vi "Set_CleanCycleHeight.vi"(8 "error in":errorcluster, 10 "CleanCycleHeight":i32, 11 "camera handle in":u64) -> (0 "error out":errorcluster, 3 "camera handle out":u64)   [LabVIEW 2014, in "PICam.lvlib"]
doc: "Controls the number of rows in a clean cycle. The default value is equal with the Y pixel size of the CCD (for example, PIXIS400: 400)."
uses:
  PICam.lvlib
  Picam32.dll
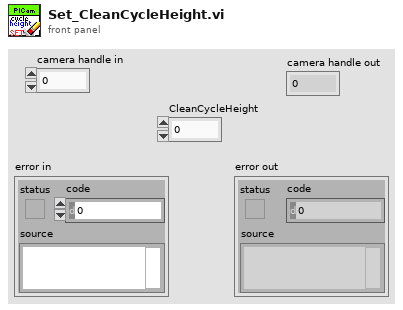
[diagram p1: front panel]
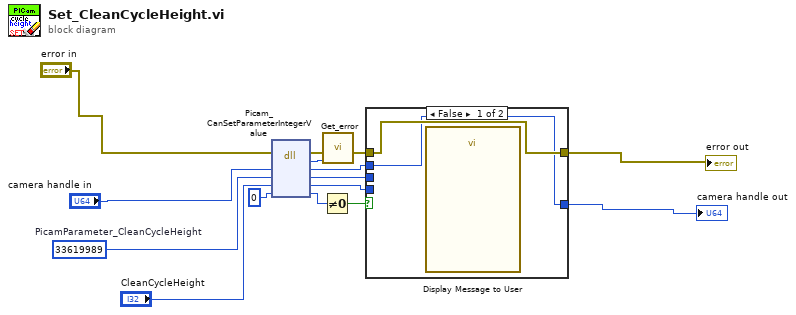
[diagram p0: block diagram]
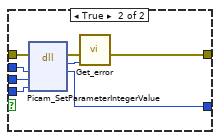
[diagram p2: hidden frame]
diagram:
  w6 = u32 33619989  # PicamParameter_CleanCycleHeight
  n1 = dll-call lib="Picam32.dll" fn="Picam_CanSetParameterIntegerValue"(error in="error in", "camera"="camera handle in", "PicamParameter"=w6, "CleanCycleHeight"="CleanCycleHeight", "bln"=0 ("CleanSerialRegister")) -> (error out=w14:errorcluster, "return type"=w15:i32, "camera"=w7:u64, "PicamParameter"=w5:u32, "CleanCycleHeight"=w10:i32, "bln"=w11:i32)  [unwired: 2 in, 1 out]
  n2 = Not Equal To 0?(x=w11) -> (x != 0?=w9:bool)
  n3 = call "Get_error.vi"("PICam_Error"=w15, "error in (no error)"=w14) -> ("error out"=w8:errorcluster)  [unwired: 9 in]
  n4 = case shown="False" w9 {
    tunnel: w10 -> [_ w23]
    tunnel: w8 -> [w17 w22]
    tunnel: w7 -> [w16 w21]
    tunnel: w5 -> [_ w20]
    tunnel: [w17 w19] -> w4
    tunnel: [w16 w18] -> w3
    frame False {
      n5 = call "Display Message to User"() -> ()  [unwired: 10 in, 2 out]
    }
    frame True {
      n6 = dll-call lib="Picam32.dll" fn="Picam_SetParameterIntegerValue"(error in=w22, "camera"=w21, "PicamParameter"=w20, "CleanCycleHeight"=w23) -> (error out=w25:errorcluster, "return type"=w24:i32, "camera"=w18:u64)  [unwired: 4 in, 1 out]
      n7 = call "Get_error.vi"("PICam_Error"=w24, "error in (no error)"=w25) -> ("error out"=w19:errorcluster)  [unwired: 9 in]
    }
  }
  "error out" <- w4
  "camera handle out" <- w3
